vi "MTM2_monitorCommand_clearErrors.vi"(8 "error in (no error)":errorcluster, 11 "command_clearErrors_Ctl":T1) -> (0 "error out":errorcluster, 2 "function return":i32, 3 "command_clearErrors_Ctl out":T1)   [LabVIEW 2018, in "SALLV_MTM2.lvlib"]
doc: "int MTM2_shm_monitorCommand_clearErrorsLV(MTM2_command_clearErrorsLV *command_clearErrors_Ctl );"
uses:
  DataTypes/command_clearErrors.ctl
  SALLV_MTM2.lvlib
  SALLV_MTM2.so
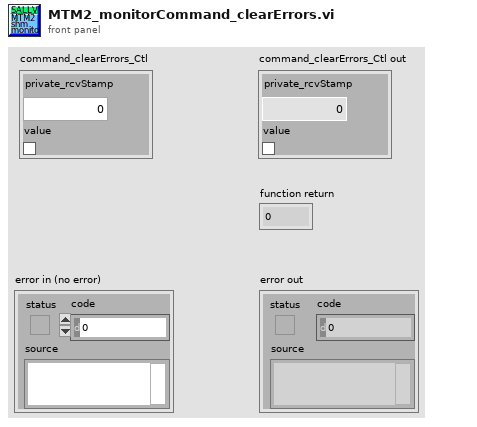
[diagram p1: front panel]
types:
  T1 = typedef "SALLV_MTM2.lvlib/command_clearErrors.ctl" = cluster{"private_rcvStamp":dbl, "value":bool}
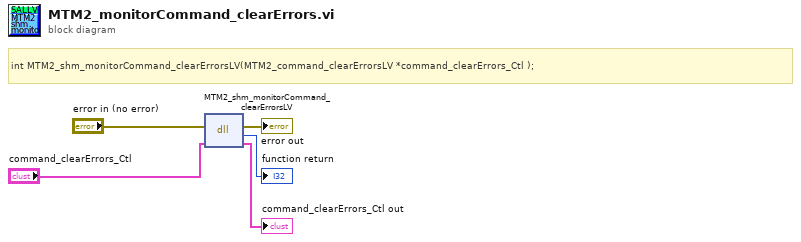
[diagram p0: block diagram]
diagram:
  # "int MTM2_shm_monitorCommand_clearErrorsLV(MTM2_command_clearErrorsLV *command_clearErrors_Ctl );"
  n1 = dll-call lib="home/ttsai/Documents/salTestLabViewApi/SALLV_MTM2/SALLV_MTM2.*" fn="MTM2_shm_monitorCommand_clearErrorsLV"(error in="error in (no error)", "command_clearErrors_Ctl"="command_clearErrors_Ctl") -> (error out=→"error out":errorcluster, →"function return":i32, "command_clearErrors_Ctl"=→"command_clearErrors_Ctl out":T1)  [unwired: 2 in, 1 out]
